vi "CalcIndicesAndLengths.vi"(9 "Index 2":i32, 10 "Index 1":i32, 11 "size(s)":i16[](array[numeric])) -> (0 "Length 2":i32, 1 "Start Index 2":i32, 2 "Length 1":i32, 3 "Start Index 1":i32)   [LabVIEW 2012]
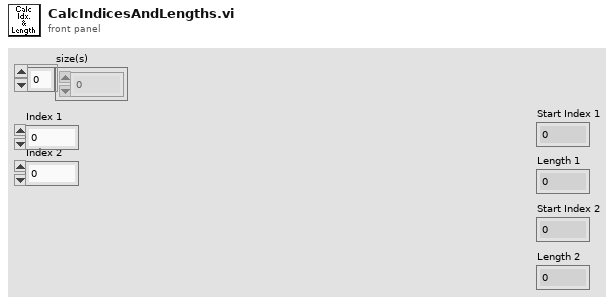
[diagram p1: front panel]
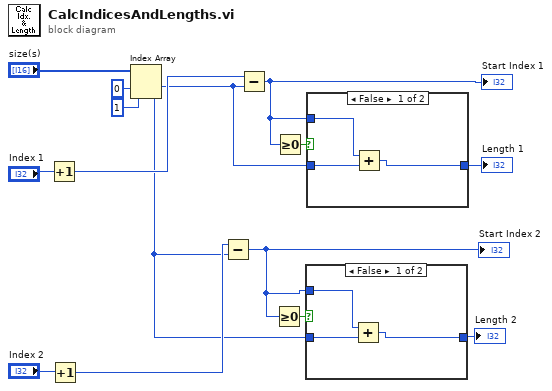
[diagram p0: block diagram]
diagram:
  n1 = Increment(x="Index 1") -> (x+1=w10:i32)
  n2 = Increment(x="Index 2") -> (x+1=w9:i32)
  n3 = Index Array(array="size(s)", index #1=0, index #2=1) -> (element #1=w7:i16, element #2=w2:i16)
  n4 = Subtract(x=w9, y=w2) -> (x-y=w3:i32)
  "Start Index 2" <- w3
  n5 = Subtract(x=w10, y=w7) -> (x-y=w5:i32)
  "Start Index 1" <- w5
  n6 = Greater Or Equal To 0?(x=w3) -> (x >= 0?=w4:bool)
  n7 = Greater Or Equal To 0?(x=w5) -> (x >= 0?=w8:bool)
  n8 = case shown="False" w4 {
    tunnel: w2 -> [w18 w19]
    tunnel: [w16 w19] -> w1
    tunnel: w3 -> [w17 _]
    frame False {
      n9 = Add(x=w17, y=w18) -> (x+y=w16:i32)
    }
    frame True {
    }
  }
  "Length 2" <- w1
  n10 = case shown="False" w8 {
    tunnel: w7 -> [w22 w23]
    tunnel: [w20 w23] -> w6
    tunnel: w5 -> [w21 _]
    frame False {
      n11 = Add(x=w21, y=w22) -> (x+y=w20:i32)
    }
    frame True {
    }
  }
  "Length 1" <- w6
